vi "NewClimb.vi"   [LabVIEW 2012]
uses:
  State_Machine_Enum.ctl
  <vilib>/Rock Robotics/WPI/Solenoid/WPI_SolenoidValue.ctl
  Sally_Dashboard_2014/DBNameEnum.ctl
  RefnameEnum.ctl
  Robot Global Data.vi
  <vilib>/Rock Robotics/WPI/Solenoid/WPI_SolenoidSetEnum.vi
types:
  T1 = typedef "State_Machine_Enum.ctl" = enum16{"Idle", "Start", "Do", "Stop", "Init"}
  T2 = typedef "WPI_SolenoidValue.ctl" = enum16{"Off", "On", "Forward", "Reverse"}
  T3 = typedef "DBNameEnum.ctl" = enum16{"AutoInstructions", "DriveLoopTime", "DriveAlignLSLeft", "DriveAlignLSRight", "Use2DriveAlign", "ClimbLS", "LauncherAngleMatches", "FrameworkVersion", "sLauncherAngle", "LauncherTargetAngle", "sLauncherRPM", "LauncherTargetRPM", "sDriveDistance", "LauncherMotorValue", "PullbackTol", "FireTol", "LauncherRPMTol", "LauncherAngleTol", "InitialWait", "WaitBetweenLaunch", "AnglePresets", "RPMPresets", "UseAngleEncoder", "UseLauncherEncoder", "UseLauncherPID", "QSWaitBeforeFire", "QSWaitBeforeRetract", "AngleForwardValue", "AngleBackwardValue", "UseClusterArray", "BackupAuto", "ReverseDriveIndicate", "HalfSpeedFactor"}
  T4 = typedef "RefnameEnum.ctl" = enum16{"FireLauncher", "Climber", "Shield", "TankDrive", "DriveEncoderL", "DriveEncoderR", "LauncherMotorRPM", "LauncherEncoderAnalog", "LauncherEncoderRPM", "ShooterLS", "DriveAlignLSLeft", "DriveAlignLSRight", "ClimbingLS", "LauncherEncoderAngle", "LauncherMotorAngle", "Gamepad1", "Gamepad2", "Compressor", "ClimbWeightSol3", "ClimbWeightSol4"}
  T5 = typedef "WPI_SolenoidDevRef.ctl" = cluster{"DevStatus":errorcluster, "Solenoid Module":T6, "Forward Solenoid Channel":T7, "Reverse Solenoid Channel":T7}
  T6 = typedef "FPGA_TypedefSolenoidModule.ctl" = enum16{"Solenoid Module 1", "Solenoid Module 2"}
  T7 = typedef "WPI_SolenoidChannel.ctl" = enum8{"Solenoid 1", "Solenoid 2", "Solenoid 3", "Solenoid 4", "Solenoid 5", "Solenoid 6", "Solenoid 7", "Solenoid 8", "Invalid"}
  T8 = typedef "WPI_DigitalInputDevRef.ctl" = cluster{"DevStatus":errorcluster, "DIO Channel":T9, "Digital Module":T10}
  T9 = typedef "FPGA_DIOChannel.ctl" = enum8{"DIO 1", "DIO 2", "DIO 3", "DIO 4", "DIO 5", "DIO 6", "DIO 7", "DIO 8", "DIO 9", "DIO 10", "DIO 11", "DIO 12", "DIO 13", "DIO 14", "Invalid"}
  T10 = typedef "FPGA_TypedefDigitalModule.ctl" = enum16{"Digital Module 1", "Digital Module 2"}
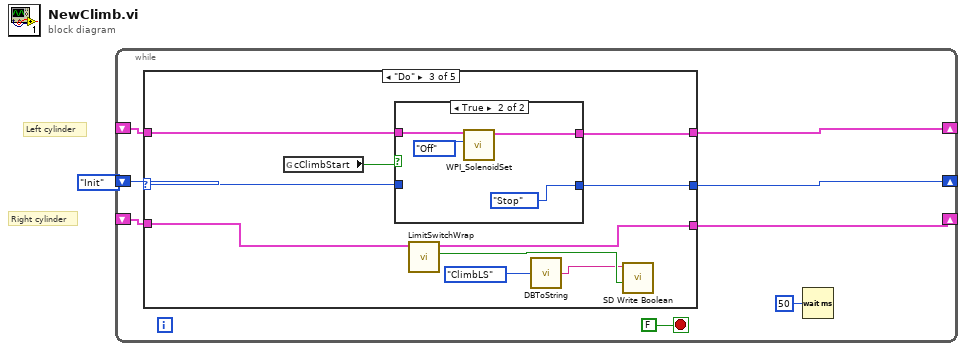
[diagram p0: block diagram]
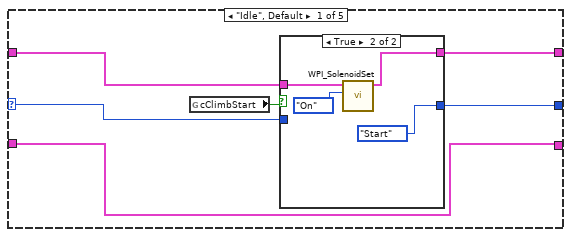
[diagram p2: hidden frame]
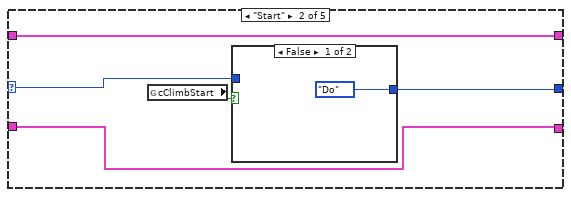
[diagram p4: hidden frame]
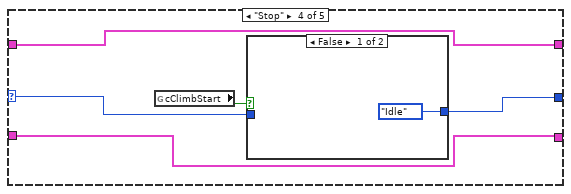
[diagram p7: hidden frame]
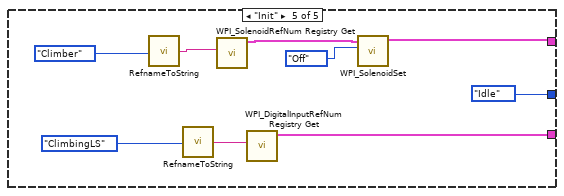
[diagram p9: hidden frame]
diagram:
  # "Right cylinder"
  # "Left cylinder"
  n1 = while {
    shift-right: [w8] -> _
    shift-left: State_Machine_Enum."Init" ("State") -> [w9]
    shift-right: [w7] -> _
    shift-left: _ -> [w6]
    shift-right: [w3] -> _
    shift-left: _ -> [w2]
    stop <- FALSE stop-if-true
    n2 = case shown="\"Do\"" w9 {
      selector: w9 -> [w11 w23 w34 w47 _]
      tunnel: [w12 w24 w35 w48 State_Machine_Enum."Idle" ("State")] -> w8
      tunnel: [w13 w26 w36 w46 w58] -> w7
      tunnel: w6 -> [w14 w26 w37 w46 _]
      tunnel: [w10 w22 w32 w45 w56] -> w3
      tunnel: w2 -> [w10 w22 w31 w45 _]
      frame "Idle", Default {
        n3 = global read "Robot Global Data.vi" "cClimbStart"() -> (w15:bool)
        n4 = case shown="True" w15 {
          tunnel: w14 -> [w16 w21]
          tunnel: [w16 w20] -> w13
          tunnel: [w17 State_Machine_Enum."Start" ("State")] -> w12
          tunnel: w11 -> [w17 _]
          frame False {
          }
          frame True {
            n5 = call-poly <vilib>:"WPI_SolenoidSet.vi"("Value"=WPI_SolenoidValue."On", "SolenoidDevRef"=w21) -> ("SolenoidDevRef"=w20:T5)  [unwired: 8 in, 1 out]
          }
        }
      }
      frame "Start" {
        n6 = global read "Robot Global Data.vi" "cClimbStart"() -> (w25:bool)
        n7 = case shown="False" w25 {
          tunnel: [State_Machine_Enum."Do" ("State") w28] -> w24
          tunnel: w23 -> [_ w28]
          frame False {
          }
          frame True {
          }
        }
      }
      frame "Do" {
        n8 = global read "Robot Global Data.vi" "cClimbStart"() -> (w38:bool)
        n9 = case shown="True" w38 {
          tunnel: w37 -> [w40 w44]
          tunnel: [w40 w43] -> w36
          tunnel: [w39 State_Machine_Enum."Stop" ("State")] -> w35
          tunnel: w34 -> [w39 _]
          frame False {
          }
          frame True {
            n10 = call-poly <vilib>:"WPI_SolenoidSet.vi"("Value"=WPI_SolenoidValue."Off", "SolenoidDevRef"=w44) -> ("SolenoidDevRef"=w43:T5)  [unwired: 8 in, 1 out]
          }
        }
        n11 = call "LimitSwitchWrap.vi"("DigitalInputDevRef"=w31) -> ("Triggered"=w33:bool, "DigitalInputDevRef 2"=w32:T8)  [unwired: 9 in]
        n12 = call "DBToString.vi"("Enum"=DBNameEnum."ClimbLS") -> ("Refname"=w30:string)
        n13 = call <vilib>:"SD Write Boolean.vi"("Boolean"=w33, "Name"=w30) -> ()  [unwired: 8 in, 2 out]
      }
      frame "Stop" {
        n14 = global read "Robot Global Data.vi" "cClimbStart"() -> (w49:bool)
        n15 = case shown="False" w49 {
          tunnel: [State_Machine_Enum."Idle" ("State") w51] -> w48
          tunnel: w47 -> [_ w51]
          frame False {
          }
          frame True {
          }
        }
      }
      frame "Init" {
        n16 = call "RefnameToString.vi"("Enum"=RefnameEnum."Climber") -> ("Refname"=w54:string)
        n17 = call "RefnameToString.vi"("Enum"=RefnameEnum."ClimbingLS") -> ("Refname"=w52:string)
        n18 = call <vilib>:"WPI_SolenoidRefNum Registry Get.vi"("refnum name"=w54) -> ("SolenoidDevRef"=w59:T5)  [unwired: 9 in, 1 out]
        n19 = call <vilib>:"WPI_DigitalInputRefNum Registry Get.vi"("refnum name"=w52) -> ("DigitalInputDevRef"=w56:T8)  [unwired: 9 in, 1 out]
        n20 = call-poly <vilib>:"WPI_SolenoidSet.vi"("Value"=WPI_SolenoidValue."Off", "SolenoidDevRef"=w59) -> ("SolenoidDevRef"=w58:T5)  [unwired: 8 in, 1 out]
      }
    }
    n21 = Wait (ms)(milliseconds to wait=u32 50) -> ()  [unwired: 1 out]
  }
